vi "HasDeviceConfiguration.vi"(8 "error in (no error)":errorcluster) -> (0 "error out":errorcluster, 3 "Has  configuration":bool)   [LabVIEW 2017, in "GlobalConfiguration.lvlib"]
uses:
  <vilib>/addons/InsightCM/Utilities/GlobalConfiguration/GlobalConfiguration.lvlib
  <vilib>/addons/PointValueMap/subVIs/Point_Read_variant.vi
  <vilib>/addons/PointValueMap/PointValueMap.lvlib
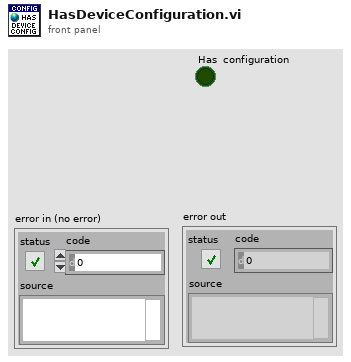
[diagram p1: front panel]
types:
  T1 = typedef "PointValueMap.lvlib/PointMap.ctl" = refnum<data-value>
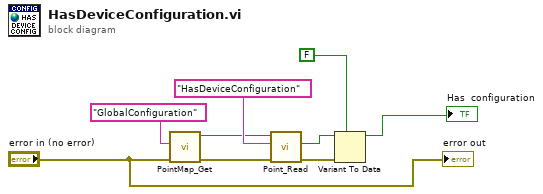
[diagram p0: block diagram]
diagram:
  n1 = call <vilib>:"PointMap_Get.vi"("error in (no error)"="error in (no error)", "Name"="GlobalConfiguration") -> ("error out"=w8:errorcluster, "Map Out"=w6:T1)  [unwired: 7 in, 1 out]
  n2 = call-poly <vilib>:"Point_Read.vi"("Error In"=w8, "Tag"="HasDeviceConfiguration" ("Name"), "Map"=w6) -> ("Error Out"=w5:errorcluster, "Found?"=w4:bool)  [unwired: 3 in, 4 out]
  n3 = Variant To Data(error in=w5, type=FALSE, Variant=w4) -> (data=→"Has  configuration":bool)  [unwired: 1 out]
  "error out" <- "error in (no error)"
